vi "Versioned Write BDX.vi"(9 "Path Stuff":T11 {"?"."Limits"."StoopidFast (fps)" min=0.0; "?"."Limits"."Jerk (fps^3)" min=0.0 step=1.0; "?"."Limits"."Accel (fps^2)" min=0.0; "?"."Limits"."Velocity (fps)" min=0.0; "?"."Overrides"."Angle Override" step=5.0; "?"."Overrides"."Velocity Override" step=5.0; "?"."Overrides"."Angular Override" step=5.0; "?"."Angular Limits"."Jerk (deg/s^3)" min=0.0 step=1.0; "?"."Angular Limits"."Accel (deg/s^2)" min=0.0; "?"."Angular Limits"."Velocity (deg/s)" min=0.0}, 10 "Filename":string, 11 "Bordeaux paths in":path) -> ()   [LabVIEW 2025]
uses:
  Types/Trajectory Data.ctl
  Types/Segment Type.ctl
  Types/Full Command Info.ctl
  Types/Single Cmd Info.ctl
  <vilib>/picture/picture.llb/imagedata.ctl
  Types/Limits.ctl
  Types/Overrides.ctl
  Types/Angluar Limits.ctl
  Types/Drive Type.ctl
  Types/Path Type.ctl
panel:
  in  "?":T12
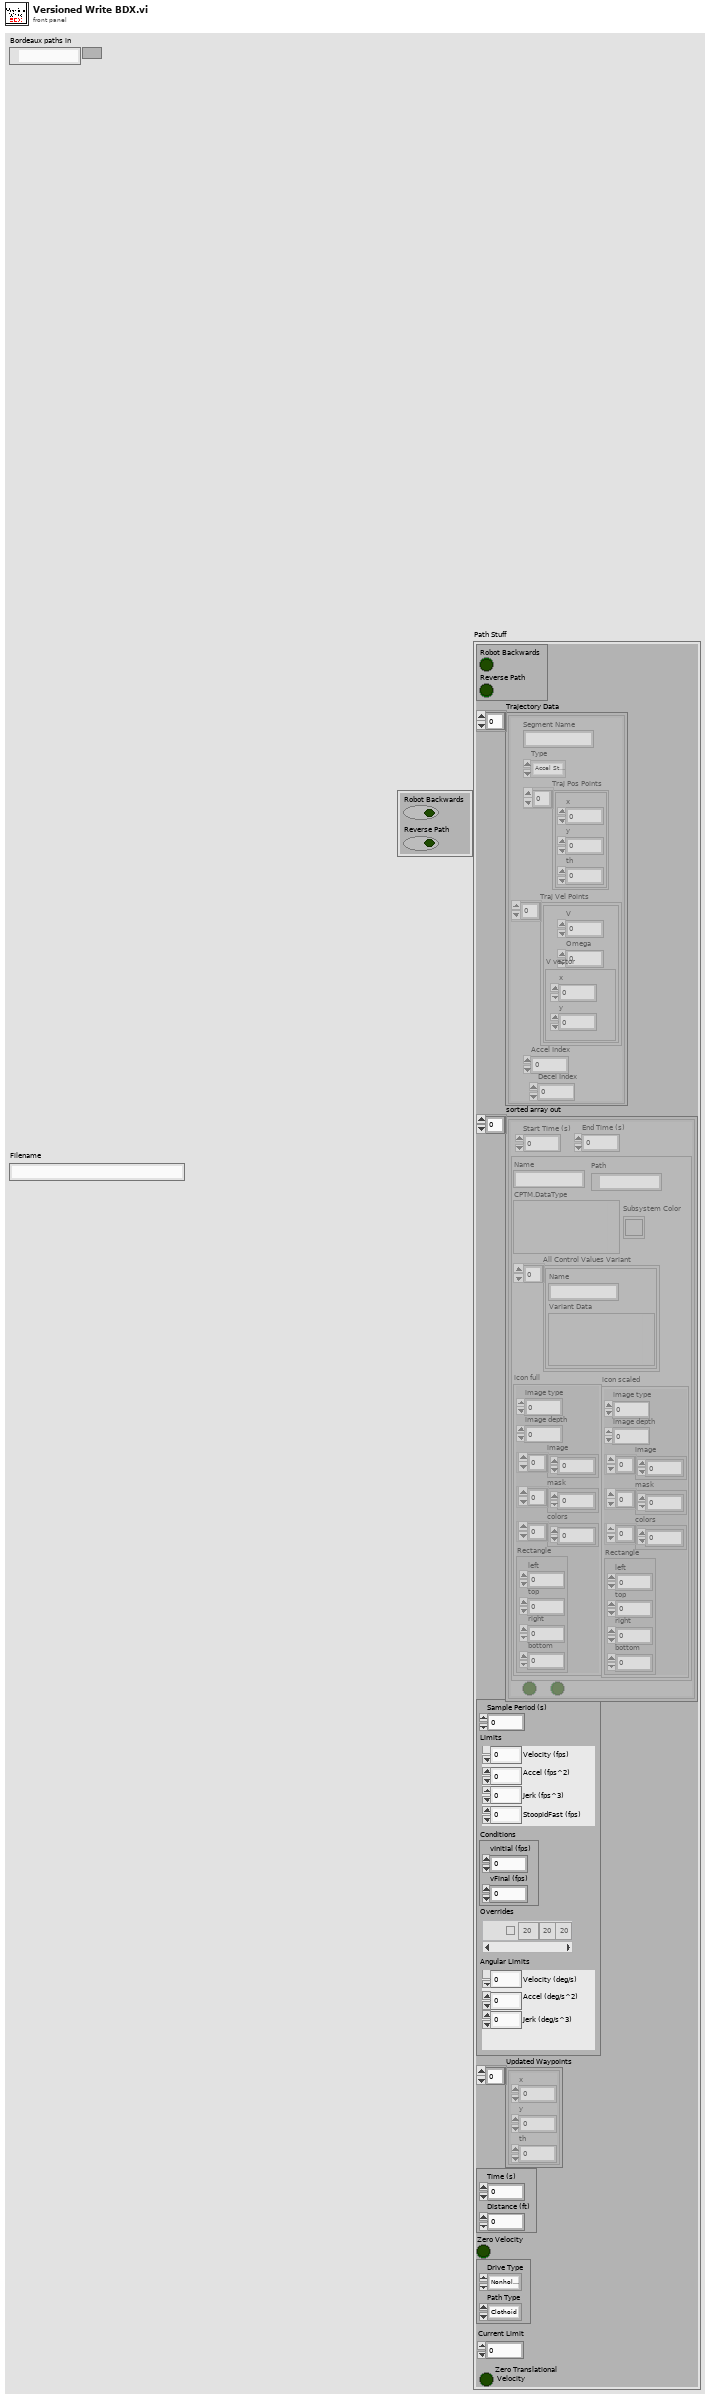
[diagram p1: front panel]
types:
  T1 = typedef "Trajectory Data.ctl" = cluster{"Segment Name":string, "Type":T2, "Traj Pos Points":cluster{"x":dbl, "y":dbl, "th":dbl}[], "Traj Vel Points":cluster{"V":dbl, "Omega":dbl, "V vector":cluster{"y":dbl, "x":dbl}}[], "Accel Index":i32, "Decel Index":i32}[]
  T2 = typedef "Segment Type.ctl" = enum16{"Accel Straight", "Const Straight", "Blend", "Circle", "Bezier"}
  T3 = typedef "Full Command Info.ctl" = cluster{"Start Time (s)":dbl, "End Time (s)":dbl, T4, "Visible":bool, "Enabled?":bool}[]
  T4 = typedef "Single Cmd Info.ctl" = cluster{"Name":string, "CPTM.DataType":variant, "All Control Values Variant":cluster{"Name":string, "Variant Data":variant}[], "icon full":T5, "icon scaled":T5, "Path":path, "Subsystem Color":u32}
  T5 = typedef "imagedata.ctl" = cluster{"image type":i32, "image depth":i32, "image":u8[], "mask":u8[], "colors":u32[], "Rectangle":cluster{"left":i16, "top":i16, "right":i16, "bottom":i16}}
  T6 = typedef "Limits.ctl" = cluster{"Velocity (fps)":dbl, "Accel (fps^2)":dbl, "Jerk (fps^3)":dbl, "StoopidFast (fps)":dbl}
  T7 = typedef "Overrides.ctl" = cluster{"Count":string, "Angular Override":dbl, "Enabled?":bool, "Velocity Override":dbl, "Angle Override":dbl}[]
  T8 = typedef "Angluar Limits.ctl" = cluster{"Velocity (deg/s)":dbl, "Accel (deg/s^2)":dbl, "Jerk (deg/s^3)":dbl}
  T9 = typedef "Drive Type.ctl" = enum16{"Nonholonomic", "Holonomic"}
  T10 = typedef "Path Type.ctl" = enum16{"Clothoid", "Bezier"}
  T11 = cluster{cluster{"Robot Backwards":bool, "Reverse Path":bool}, "Trajectory Data":T1, "sorted array out":T3, cluster{"Sample Period (s)":dbl, "Limits":T6, "Conditions":cluster{"vInitial (fps)":dbl, "vFinal (fps)":dbl}, "Overrides":T7, "Angular Limits":T8}, "Updated Waypoints":cluster{"x":dbl, "y":dbl, "th":dbl}[], cluster{"Time (s)":dbl, "Distance (ft)":dbl}, "Zero Velocity":bool, cluster{"Drive Type":T9, "Path Type":T10}, "Current Limit":dbl, "Zero Translational\n Velocity":bool}
  T12 = cluster{"Robot Backwards":bool, "Reverse Path":bool}
  T13 = cluster{"Sample Period (s)":dbl, "Limits":T6, "Conditions":cluster{"vInitial (fps)":dbl, "vFinal (fps)":dbl}, "Overrides":T7, "Angular Limits":T8}
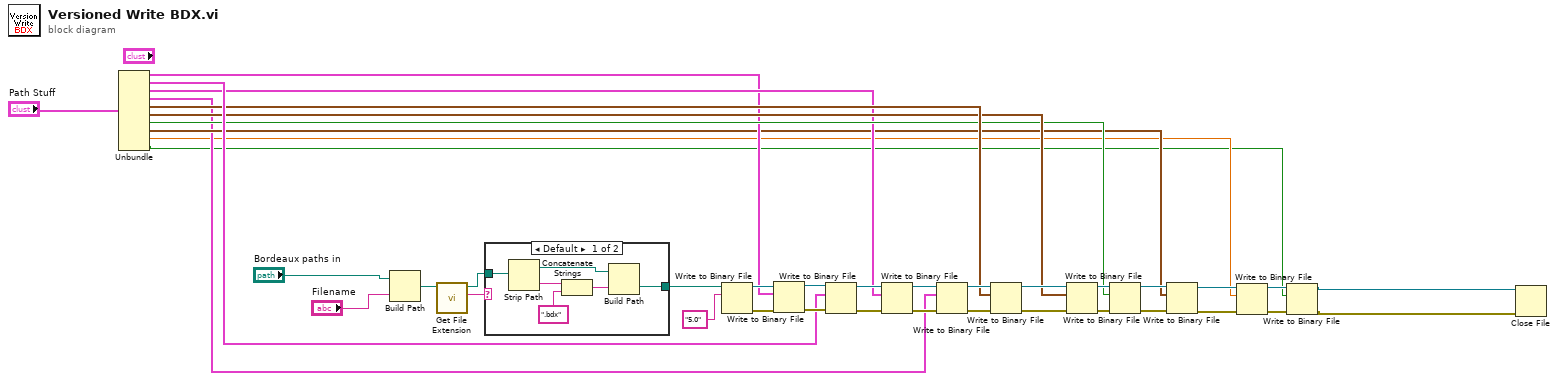
[diagram p0: block diagram]
diagram:
  n1 = Unbundle("Path Stuff") -> (w14:T12, "Trajectory Data"=w19:T1, "sorted array out"=w15:T3, w10:T13, "Updated Waypoints"=w18:cluster{"x":dbl, "y":dbl, "th":dbl}[], w17:cluster{"Time (s)":dbl, "Distance (ft)":dbl}, "Zero Velocity"=w16:bool, w11:cluster{"Drive Type":T9, "Path Type":T10}, "Current Limit"=w7:dbl, "Zero Translational\n Velocity"=w3:bool)
  n2 = Build Path(base path="Bordeaux paths in", name or relative path="Filename") -> (appended path=w37:path)
  n3 = call <vilib>:"Get File Extension.vi"("file"=w37) -> ("lowercase file extension"=w38:string, "dup file"=w39:path)  [unwired: 6 in, 3 out]
  n4 = case shown="Default" w38 {
    tunnel: w39 -> [w45 w47]
    tunnel: [w42 w47] -> w40
    frame Default {
      n5 = Strip Path(path=w45) -> (stripped path=w43:path, name=w44:string)
      n6 = Concatenate Strings(w44, ".bdx") -> (w41:string)
      n7 = Build Path(base path=w43, name or relative path=w41) -> (appended path=w42:path)
    }
    frame "bdx" {
    }
  }
  n8 = Write to Binary File(file (use dialog)=w40, data="5.0") -> (refnum out=w22:refnum<file>, error out=w28:errorcluster)  [unwired: 4 in, 1 out]
  n9 = Write to Binary File(file (use dialog)=w22, data=w14, error in=w28) -> (refnum out=w24:refnum<file>, error out=w29:errorcluster)  [unwired: 3 in, 1 out]
  n10 = Write to Binary File(file (use dialog)=w24, data=w19, error in=w29) -> (refnum out=w25:refnum<file>, error out=w30:errorcluster)  [unwired: 3 in, 1 out]
  n11 = Write to Binary File(file (use dialog)=w25, data=w15, error in=w30) -> (refnum out=w26:refnum<file>, error out=w31:errorcluster)  [unwired: 3 in, 1 out]
  n12 = Write to Binary File(file (use dialog)=w26, data=w10, error in=w31) -> (refnum out=w20:refnum<file>, error out=w32:errorcluster)  [unwired: 3 in, 1 out]
  n13 = Write to Binary File(file (use dialog)=w20, data=w18, error in=w32) -> (refnum out=w23:refnum<file>, error out=w33:errorcluster)  [unwired: 3 in, 1 out]
  n14 = Write to Binary File(file (use dialog)=w23, data=w17, error in=w33) -> (refnum out=w27:refnum<file>, error out=w34:errorcluster)  [unwired: 3 in, 1 out]
  n15 = Write to Binary File(file (use dialog)=w27, data=w16, error in=w34) -> (refnum out=w13:refnum<file>, error out=w12:errorcluster)  [unwired: 3 in, 1 out]
  n16 = Write to Binary File(file (use dialog)=w13, data=w11, error in=w12) -> (refnum out=w8:refnum<file>, error out=w6:errorcluster)  [unwired: 3 in, 1 out]
  n17 = Write to Binary File(file (use dialog)=w8, data=w7, error in=w6) -> (refnum out=w4:refnum<file>, error out=w5:errorcluster)  [unwired: 3 in, 1 out]
  n18 = Write to Binary File(file (use dialog)=w4, data=w3, error in=w5) -> (refnum out=w2:refnum<file>, error out=w1:errorcluster)  [unwired: 3 in, 1 out]
  n19 = Close File(refnum=w2, error in=w1) -> ()  [unwired: 2 out]
